vi "InsertionSortTest.vi"() -> ()   [LabVIEW 2020]
uses:
  Typedef/Record.ctl
panel:
  out "Records Sorted":T1[](array[typedef])
  in  "Records In":T1[](array[typedef])=[{"raw data"=[], "ID"=0, "Size (bytes)"=0, "Timestamp"=12}, {"raw data"=[], "ID"=0, "Size (bytes)"=0, "Timestamp"=5}, {"raw data"=[], "ID"=0, "Size (bytes)"=0, "Timestamp"=3}, {"raw data"=[], "ID"=0, "Size (bytes)"=0, "Timestamp"=20}, {"raw data"=[], "ID"=0, "Size (bytes)"=0, "Timestamp"=8}, {"raw data"=[], "ID"=0, "Size (bytes)"=0, "Timestamp"=1}, {"raw data"=[], "ID"=0, "Size (bytes)"=0, "Timestamp"=8}, {"raw data"=[], "ID"=0, "Size (bytes)"=0, "Timestamp"=9}, {"raw data"=[], "ID"=0, "Size (bytes)"=0, "Timestamp"=12}, {"raw data"=[], "ID"=0, "Size (bytes)"=0, "Timestamp"=15}, {"raw data"=[], "ID"=0, "Size (bytes)"=0, "Timestamp"=3}]
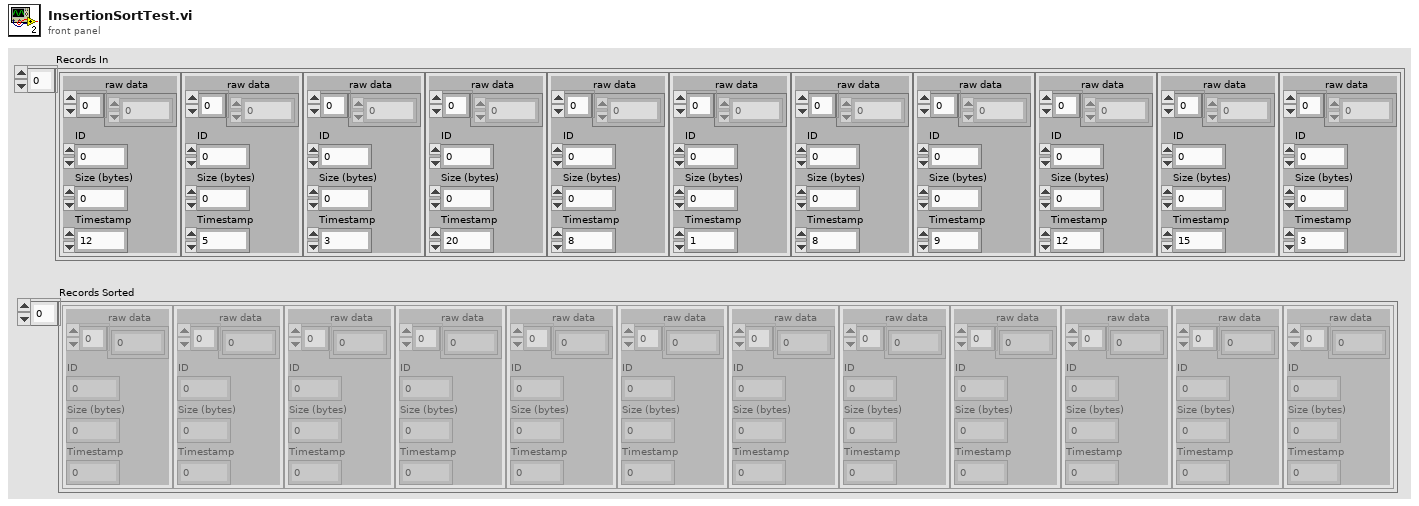
[diagram p1: front panel]
types:
  T1 = typedef "Record.ctl" = cluster{"raw data":u8[], "ID":u32, "Size (bytes)":u32, "Timestamp":u64}
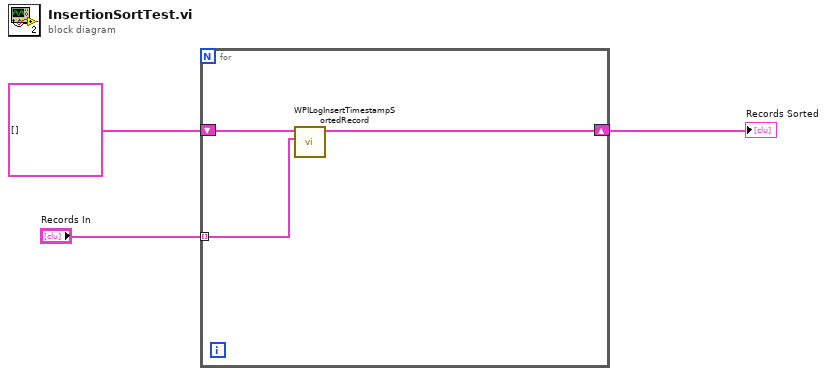
[diagram p0: block diagram]
diagram:
  n1 = for {
    shift-right: [w5] -> w2
    shift-left: T1[] [] ("Records") -> [w6]
    tunnel: "Records In" -> [w4] mode=indexing
    n2 = call "WPILogInsertTimestampSortedRecord.vi"("Record"=w4, "Records"=w6) -> ("Array"=w5:T1[])  [unwired: 9 in]
  }
  "Records Sorted" <- w2
